vi "PRO_Check_LevelV1.vi"(8 "Results In":T1 {"Resistor 2" format="%.1f"; "Drain" format="%.3f"; "Resistor" format="%.1f"; "Fill" format="%.3f"}, 9 "Level In":T4, 11 "ChA Spec RNG In":T5) -> (0 "Results Out":T1 {"Resistor 2" format="%.1f"; "Drain" format="%.3f"; "Resistor" format="%.1f"; "Fill" format="%.3f"}, 1 "Bad Switch":bool, 2 "Switched Code":i32=4, 3 "Err Num":i32)   [LabVIEW 2024]
uses:
  Control Definitions/Def Spec RNG.ctl
  Control Definitions/Ded LUT_Status.ctl
  Control Definitions/Def_LevelSwitched.ctl
  Control Definitions/Def_ATPStatus.ctl
  Control Definitions/DEF_ Results3.ctl
  Control Definitions/DEF_Results1D.ctl
panel:
  out "ChA/!ChB":bool
  out "Boolean":bool
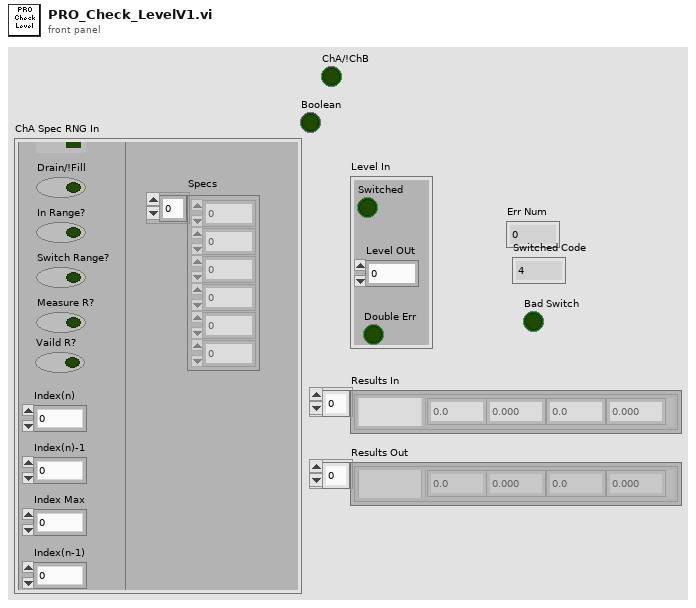
[diagram p1: front panel]
types:
  T1 = typedef "DEF_Results1D.ctl" = T2[]
  T2 = typedef "DEF_ Results3.ctl" = cluster{"Fill":dbl, "Status":T3, "Resistor":dbl, "Drain":dbl, "Resistor 2":dbl}
  T3 = typedef "Def_ATPStatus.ctl" = i16
  T4 = typedef "Def_LevelSwitched.ctl" = cluster{"Switched":bool, "Level OUt":dbl, "Double Err":bool}
  T5 = typedef "Def Spec RNG.ctl" = cluster{"Specs":dbl[], "LUT Status":T6}
  T6 = typedef "Ded LUT_Status.ctl" = cluster{"ChA/!ChB":bool, "Drain/!Fill":bool, "In Range?":bool, "Switch Range?":bool, "Measure R?":bool, "Vaild R?":bool, "Index(n)":i32, "Index(n)-1":i32, "Index Max":i32, "Index(n-1)":i32}
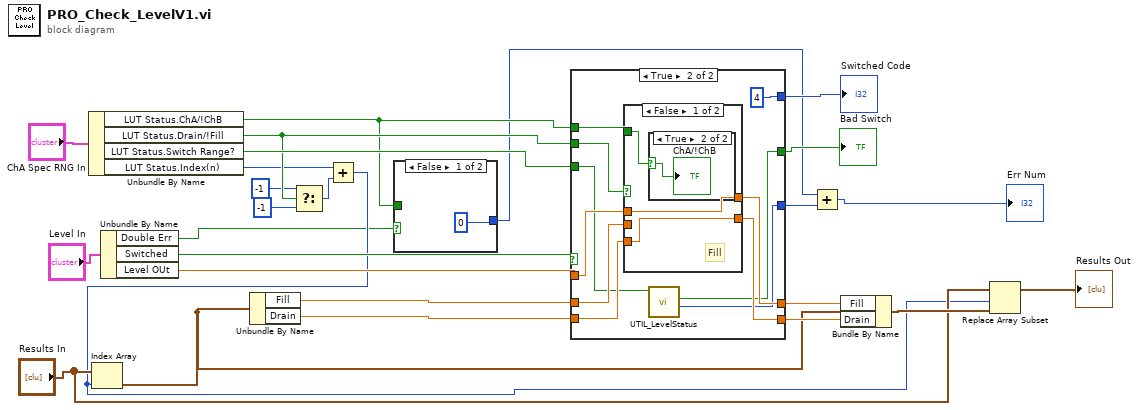
[diagram p0: block diagram]
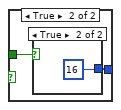
[diagram p2: hidden frame]
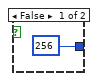
[diagram p3: hidden frame]
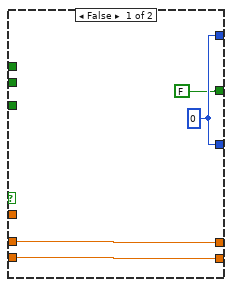
[diagram p4: hidden frame]
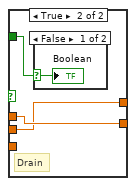
[diagram p6: hidden frame]
diagram:
  n1 = Unbundle By Name("ChA Spec RNG In") -> ("LUT Status.ChA/!ChB"=w5:bool, "LUT Status.Drain/!Fill"=w11:bool, "LUT Status.Switch Range?"=w19:bool, "LUT Status.Index(n)"=w6:i32)
  n2 = Unbundle By Name("Level In") -> ("Double Err"=w4:bool, "Switched"=w16:bool, "Level OUt"=w20:dbl)
  n3 = Select(t=-1, s=w11, f=-1) -> (s? t:f=w7:i32)
  n4 = Add(x=w6, y=w7) -> (x+y=w8:i32)
  n5 = Index Array(array="Results In", index=w8) -> (element=w15:T2)
  n6 = Unbundle By Name(w15) -> ("Fill"=w23:dbl, "Drain"=w24:dbl)
  n7 = case shown="False" w4 {
    tunnel: w5 -> [_ w29]
    tunnel: [0 w28] -> w1
    frame False {
    }
    frame True {
      n8 = case shown="True" w29 {
        tunnel: [256 16] -> w28
        frame False {
        }
        frame True {
        }
      }
    }
  }
  n9 = case shown="True" w16 {
    tunnel: w23 -> [w35 w46]
    tunnel: w24 -> [w34 w45]
    tunnel: w20 -> [_ w44]
    tunnel: [w34 w43] -> w25
    tunnel: [w35 w42] -> w26
    tunnel: w19 -> [_ w38]
    tunnel: w5 -> [_ w40]
    tunnel: [w33 w36] -> w3
    tunnel: w11 -> [_ w41]
    tunnel: [w33 4] -> w18
    tunnel: [FALSE w37] -> w17
    frame False {
      w33 = 0
    }
    frame True {
      n10 = case shown="False" w41 {
        tunnel: w46 -> [_ w52]
        tunnel: w45 -> [w48 _]
        tunnel: w44 -> [w49 w53]
        tunnel: [w48 w53] -> w43
        tunnel: [w49 w52] -> w42
        tunnel: w40 -> [w47 w51]
        frame False {
          # "Fill"
          n11 = case shown="True" w47 {
            selector: w47 -> [_ w50]
            frame False {
            }
            frame True {
              "ChA/!ChB" <- w50
            }
          }
        }
        frame True {
          # "Drain"
          n12 = case shown="False" w51 {
            selector: w51 -> [w54 _]
            frame False {
              "Boolean" <- w54
            }
            frame True {
            }
          }
        }
      }
      n13 = call "UTIL_LevelStatus.vi"("Good!Bad"=w38) -> ("Err Num"=w36:u32, "Bad Switch"=w37:bool)  [unwired: 8 in, 1 out]
    }
  }
  "Switched Code" <- w18
  "Bad Switch" <- w17
  n14 = Add(x=w1, y=w3) -> (x+y=→"Err Num":u32)
  n15 = Bundle By Name(cluster=w15, "Fill"=w26, "Drain"=w25) -> (w14:T2)
  n16 = Replace Array Subset(array="Results In", new element=w14, index=w8) -> (→"Results Out":T1)
